vi "Tear Down.vi"(8 "error in (no error)":errorcluster, 11 "Terminal Timeout in":refnum<class "Terminal Timeout.lvclass">) -> (0 "error out":errorcluster, 3 "Terminal Timeout out":refnum<class "Terminal Timeout.lvclass">)   [LabVIEW 2016, in "CLD Exam - ATM.lvlib" / "Terminal Timeout.lvclass"]
uses:
  Terminal Timeout.lvclass
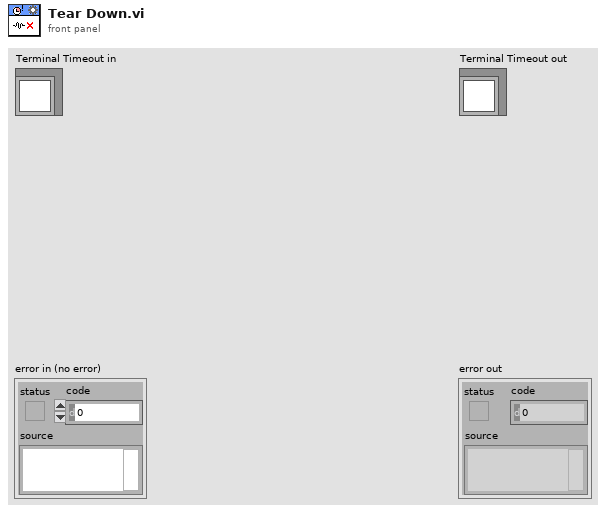
[diagram p1: front panel]
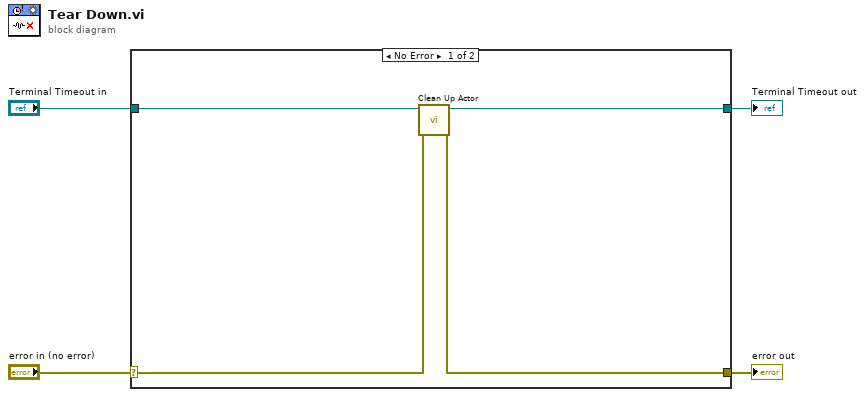
[diagram p0: block diagram]
diagram:
  n1 = case shown="No Error" "error in (no error)" {
    selector: "error in (no error)" -> [w6 w10]
    tunnel: [w5 w10] -> w3
    tunnel: [w7 w9] -> w1
    tunnel: "Terminal Timeout in" -> [w8 w9]
    frame No Error {
      n2 = call-dynamic "Clean Up Actor.vi"("error in (no error)"=w6, "Terminal Timeout in"=w8) -> ("error out"=w5:errorcluster, "Terminal Timeout out"=w7:refnum<class "Terminal Timeout.lvclass">)  [unwired: 8 in]
    }
    frame Error {
    }
  }
  "error out" <- w3
  "Terminal Timeout out" <- w1
